vi "VI Tree - comparison__ogtk.vi"   [LabVIEW 2009]
uses:
  Variant Changed__ogtk.vi
panel:
  # "[OpenG VI Tags] ***Do Not Remove***"
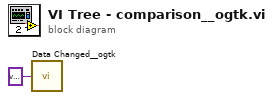
[diagram p0: block diagram]
diagram:
  n1 = call-poly "Data Changed__ogtk.vi"("Variant"=variant) -> ()  [unwired: 1 out]
